vi "TIO Form Packet.vi"(9 "Routing":string, 10 "Type":T1(ring)=enum."RPC Request", 11 "Payload":string="Q\u0017\b€dev.name") -> (3 "String out":string)   [LabVIEW 2017]
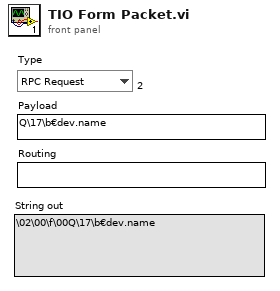
[diagram p1: front panel]
types:
  T1 = enum8{"Invalid", "Log", "RPC Request", "RPC Reply", "RPC Error", "Stream Description", "User"}
  T2 = enum16{"big-endian, network order", "native, host order", "little-endian"}
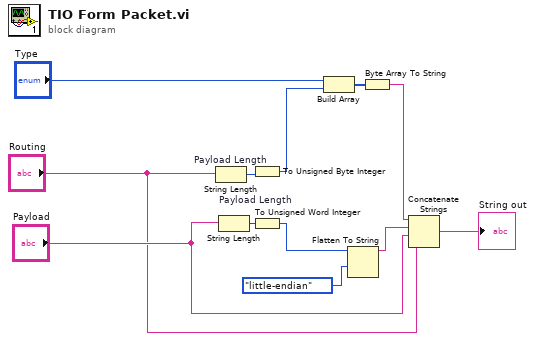
[diagram p0: block diagram]
diagram:
  n1 = String Length "Payload Length"(string="Routing") -> (length=w5:i32)
  n2 = String Length "Payload Length"(string="Payload") -> (length=w7:i32)
  n3 = To Unsigned Byte Integer(number=w5) -> (unsigned 8bit integer=w4:u8)
  n4 = To Unsigned Word Integer(number=w7) -> (unsigned 16bit integer=w9:u16)
  n5 = Build Array("Type", w4) -> (w3:u8[])
  n6 = Flatten To String(anything=w9, byte order (0:big-endian, network order)=T2."little-endian") -> (data string=w8:string)  [unwired: 2 in, 2 out]
  n7 = Byte Array To String(unsigned byte array=w3) -> (string=w2:string)
  n8 = Concatenate Strings(w2, w8, "Payload", "Routing") -> (→"String out":string)
